vi "PH_ImageStatistician.contents.vi"   [LabVIEW 2014, in "PH_ImageStatistician.lvlib"]
doc: "This class is forseen to collect data from the PH_ImageOperator class to get statistical values.\n\nThis class is part of the PHELIX user layer."
uses:
  PH_ImageStatistician.lvlib
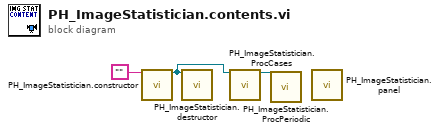
[diagram p0: block diagram]
diagram:
  n1 = call "PH_ImageStatistician.constructor.vi"("name"="") -> ("i ref out"=w2:refnum<vi>)  [unwired: 16 in, 2 out]
  n2 = call "PH_ImageStatistician.destructor.vi"("i ref in"=w2) -> ()  [unwired: 18 in, 1 out]
  n3 = call "PH_ImageStatistician.ProcCases.vi"("i ref in"=w2) -> ("i ref out"=w1:refnum<vi>)  [unwired: 16 in, 2 out]
  n4 = call "PH_ImageStatistician.ProcPeriodic.vi"("i ref in"=w1) -> ()  [unwired: 16 in, 3 out]
  n5 = call "PH_ImageStatistician.panel.vi"() -> ()  [unwired: 19 in, 1 out]
